vi "continous to paused.vi"(7 "Device model":string, 8 "error in (no error)":errorcluster, 9 "Motor control":T1, 10 "Acq args":T2, 11 "Resolution":dbl) -> (0 "error out":errorcluster, 3 "Acq arrgs out":T4)   [LabVIEW 2020]
uses:
  controls/Motor direction ---typedef.ctl
  controls/Paused acquisition ---argument.ctl
  Controls/Motor controls---typedef.ctl
  controls/Continuous acquisition ---argument.ctl
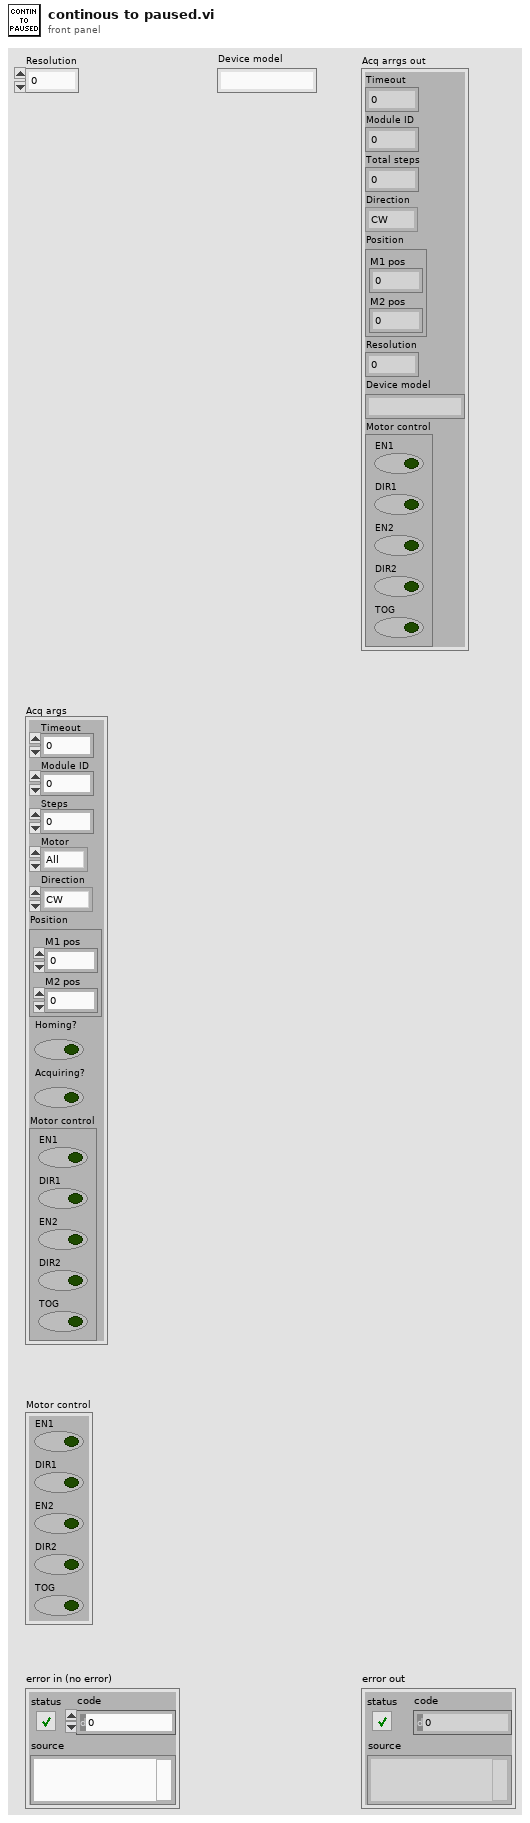
[diagram p1: front panel]
types:
  T1 = typedef "Motor controls---typedef.ctl" = cluster{"EN1":bool, "DIR1":bool, "EN2":bool, "DIR2":bool, "TOG":bool}
  T2 = typedef "Continuous acquisition ---argument.ctl" = cluster{"Timeout":i32, "Module ID":i32, "Steps":i32, "Motor":enum16{"All", "M1", "M2"}, "Direction":T3, "Position":cluster{"M1 pos":dbl, "M2 pos ":dbl}, "Homing?":bool, "Acquiring?":bool, "Motor control":T1}
  T3 = typedef "Motor direction ---typedef.ctl" = enum16{"CW", "CCW"}
  T4 = typedef "Paused acquisition ---argument.ctl" = cluster{"Timeout":i32, "Module ID":i32, "Total steps":i32, "Direction":T3, "Position":cluster{"M1 pos":dbl, "M2 pos ":dbl}, "Resolution":dbl, "Device model":string, "Motor control":T1}
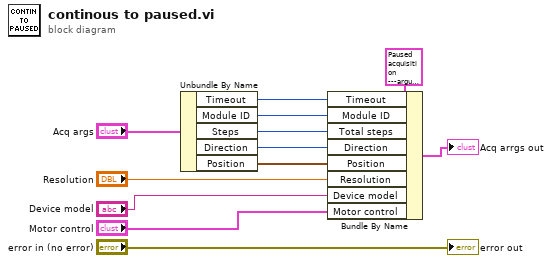
[diagram p0: block diagram]
diagram:
  n1 = Unbundle By Name("Acq args") -> ("Timeout"=w9:i32, "Module ID"=w8:i32, "Steps"=w7:i32, "Direction"=w6:T3, "Position"=w5:cluster{"M1 pos":dbl, "M2 pos ":dbl})
  n2 = Bundle By Name(cluster=T4 {"Timeout"=0, "Module ID"=0, "Total steps"=0, "Direction"=enum."CW", "Position"={"M1 pos"=0.0, "M2 pos "=0.0}, "Resolution"=0.0, "Device model"="", "Motor control"={"EN1"=FALSE, "DIR1"=FALSE, "EN2"=FALSE, "DIR2"=FALSE, "TOG"=FALSE}} ("event data"), "Timeout"=w9, "Module ID"=w8, "Total steps"=w7, "Direction"=w6, "Position"=w5, "Resolution"="Resolution", "Device model"="Device model", "Motor control"="Motor control") -> (→"Acq arrgs out":T4)
  "error out" <- "error in (no error)"
